vi "Stop Core.vi"(10 "final error code":i32, 11 "H3611i Actor in":refnum<class "H3611i Actor.lvclass">) -> (3 "H3611i Actor out":refnum<class "H3611i Actor.lvclass">)   [LabVIEW 2018, in "H3611i.lvlib" / "H3611i Actor.lvclass"]
doc: "In addition to the following, this method also sends a message to the monitor to notify it that the actor has stopped execution.\n\n(<B>Filename</B>: Actor Framework.lvlib:Actor.lvclass:Stop Core.vi)\n\nDefines what the actor does before it stops. Use the <B>final error code</B> input to determine whether the actor shut down in response to an error.\n\nBy default, this method does nothing. A descendant class may override it to define behavior, such as shutting down any processes the actor initiated in its override of the Actor Core method.\n\nCopyright: MGI\nAuthored by: Derek Trepanier"
uses:
  H3611i Actor.lvclass
  C:/Users/dev/Documents/CODE/LabVIEW/microwaveverify/trunk/MWWL Verification/Sensor Actor/Sensor/Sensor.lvclass
  H3611i Actor.lvclass/H3611i Actor.ctl
  Sensor Actor/Sensor/Sensor.lvclass
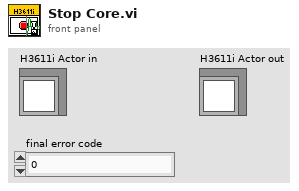
[diagram p1: front panel]
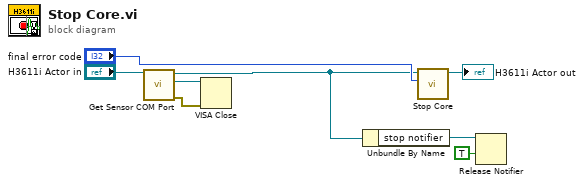
[diagram p0: block diagram]
diagram:
  n1 = call "Get Sensor COM Port.vi"("Sensor in"="H3611i Actor in") -> ("error out"=w4:errorcluster, "COM Port"=w5:refnum<visa-resource-name>, "Sensor out"=w2:refnum<class "H3611i Actor.lvclass">)  [unwired: 8 in]
  n2 = VISA Close(VISA resource name=w5, error in (no error)=w4) -> ()  [unwired: 1 out]
  n3 = Unbundle By Name(w2) -> ("stop notifier"=w1:refnum<notifier>)
  n4 = call-parent "Stop Core.vi"("final error code"="final error code", "Sensor in"=w2) -> ("Sensor out"=→"H3611i Actor out":refnum<class "H3611i Actor.lvclass">)  [unwired: 9 in]
  n5 = Release Notifier(notifier=w1, force destroy? (F)=TRUE) -> ()  [unwired: 1 in, 3 out]
